vi "filter channels by data type.vi"(8 "error in (no error)":errorcluster, 10 "data type":T1, 11 "channels in":refnum<class "TBM channel.lvclass">[](array[class])) -> (0 "error out":errorcluster, 3 "filtered channels out":refnum<class "TBM channel.lvclass">[](array[class]))   [LabVIEW 2014, in "Shared Memory configuration.lvclass"]
uses:
  Shared Memory configuration.lvclass
  <vilib>/NI/Tag Bus Module Framework/channel/TBM channel.lvclass
  <vilib>/NI/Tag Bus/tag/Data Type.ctl
  <vilib>/NI/Tag Bus/tag/tag descriptor.lvclass/tag descriptor.ctl
  <vilib>/NI/Tag Bus/tag/tag descriptor.lvclass
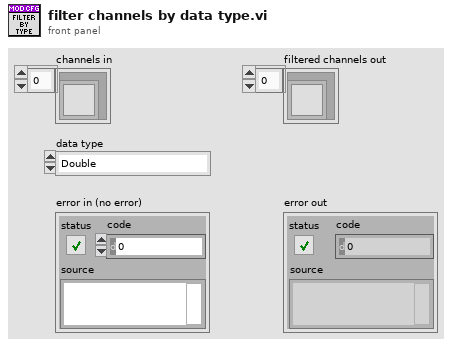
[diagram p1: front panel]
types:
  T1 = typedef "tag bus.lvlib/tag descriptor.lvclass/Data Type.ctl" = enum16{"Double", "Single", "I64", "I32", "I16", "I8", "U64", "U32", "U16", "U8", "Boolean", "String", "Array of Double", "Array of Single", "Array of I64", "Array of I32", "Array of I16", "Array of I8", "Array of U64", "Array of U32", "Array of U16", "Array of U8", "Array of Boolean", "Array of String"}
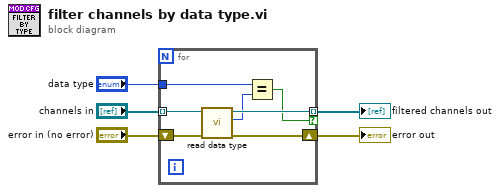
[diagram p0: block diagram]
diagram:
  n1 = for {
    shift-right: [w9] -> w2
    shift-left: "error in (no error)" -> [w11]
    tunnel: "data type" -> [w12]
    tunnel: "channels in" -> [w10] mode=indexing
    tunnel: [w8] -> w3 mode=indexing if=w6
    n2 = call <vilib>:"read data type.vi"("error in"=w11, "system tag in"=w10) -> ("error out"=w9:errorcluster, "data type"=w7:T1, "system tag out"=w8:refnum<class "TBM channel.lvclass">)  [unwired: 7 in]
    n3 = Equal?(x=w12, y=w7) -> (x = y?=w6:bool)
  }
  "filtered channels out" <- w3
  "error out" <- w2
